vi "Close.vi"(8 "error in":errorcluster) -> ()   [LabVIEW 2014, in "Elevator System.lvlib"]
uses:
  Elevator System.lvlib
  Typedef/MessageType.ctl
  Typedef/Commands.ctl
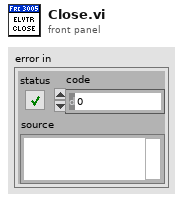
[diagram p1: front panel]
types:
  T1 = typedef "Elevator System.lvlib/Commands.ctl" = enum16{"Home", "Stack", "Pickup", "Score", "Cycle", "Stop", "Manual Open", "Manual Close", "Manual Up", "Manual Down", "Gripper RC", "Gripper Cycle", "Wait On Gripper", "Wait On Elevator"}
  T2 = typedef "Elevator System.lvlib/MessageType.ctl" = cluster{"Name":T1, "Data":variant}
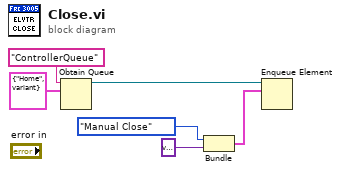
[diagram p0: block diagram]
diagram:
  n1 = Obtain Queue(name (unnamed)="ControllerQueue", element data type=T2 {"Name"=enum."Home", "Data"=variant} ("Message")) -> (queue out=w6:refnum<queue>)  [unwired: 3 in, 2 out]
  n2 = Bundle("Name"=Commands."Manual Close", variant) -> (w4:cluster{"Name":T1, variant})  [unwired: 1 in]
  n3 = Enqueue Element(queue=w6, element=w4) -> ()  [unwired: 2 in, 3 out]
